vi "Periodic Tasks.vi"(8 "error in":errorcluster) -> ()   [LabVIEW 2012]
doc: "This VI runs in parallel to other tasks. It can contain as many user-defined periodic loops as you need. These can carry out PID or other sorts of timed response."
uses:
  <vilib>/Rock Robotics/SystemInterfaces/Utilities/FPGA_UtilitiesLED Source.ctl
  <vilib>/Rock Robotics/SystemInterfaces/Utilities/FPGA_UtilitiesLED State.ctl
  <vilib>/Rock Robotics/WPI/Compressor/WPI_CompressorGetSetRefNum.vi
  Robot Global Data.vi
  <vilib>/Rock Robotics/WPI/Joystick/WPI_JoystickGetSetRefNum.vi
  <vilib>/Rock Robotics/WPI/RobotDrive/WPI_RobotDriveGetSetRefNum.vi
panel:
  out "Current angle (deg) Right":dbl(knob) scale=0.0..360.0
  out "Distance (in) Right":dbl
  out "Revolutions Right":dbl
  out "Encoder Rate (in/sec) Right":dbl
  out "Encoder Status Right":string
  out "Encoder Direction Right":string
  out "Current angle (deg) Left":dbl(knob) scale=0.0..360.0
  out "Distance (in) Left":dbl
  out "Revolutions Left":dbl
  out "Encoder Rate (in/sec) Left":dbl
  out "Encoder Status Left":string
  out "Encoder Direction Left":string
  in  "Wheel dia. (in)":dbl=6.0
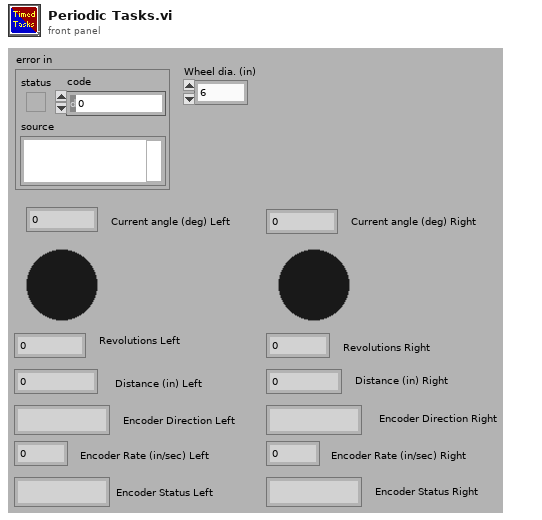
[diagram p1: front panel]
types:
  T1 = typedef "WPI_JoystickDevRef.ctl" = cluster{"Device":T2}
  T2 = typedef "WPI_JoystickDeviceEnum.ctl" = enum16{"USB 1", "USB 2", "USB 3", "USB 4", "Kinect 1", "Kinect 2"}
  T3 = typedef "WPI_RobotDriveDevRef.ctl" = cluster{"DevStatus":errorcluster, "Motors[]":T4[], "Square Inputs":bool, "Max Output":dbl, "Isochronous":bool}
  T4 = typedef "WPI_MotorControlDeviceRef.ctl" = cluster{"DeviceStatus":errorcluster, "Type":enum16{"PWM", "CAN"}, "PWM":cluster{"Digital Module":T5, "PWM Channel":T6, "DeadBand":T7}, "CAN":cluster{"Device Number":u8, "Control Mode":T8, "Semaphore":T9, "Max Vout":dbl}, "Invert":bool, "TransformRef":T10, "InvTransformRef":T10}
  T5 = typedef "FPGA_TypedefDigitalModule.ctl" = enum16{"Digital Module 1", "Digital Module 2"}
  T6 = typedef "FPGA_DIOPWMChannel.ctl" = enum8{"PWM 1", "PWM 2", "PWM 3", "PWM 4", "PWM 5", "PWM 6", "PWM 7", "PWM 8", "PWM 9", "PWM 10", "Invalid"}
  T7 = typedef "WPI_PWMDeadband.ctl" = cluster{"Name":string, "maxPositivePwm":i32, "minPositivePwm":i32, "centerPwm":i32, "maxNegativePwm":i32, "minNegativePwm":i32, "angularRange":u16}
  T8 = typedef "WPI_CANJaguar_ControlMode.ctl" = enum8{"Percent VBus", "Current", "Speed", "Position", "Voltage"}
  T9 = typedef "Semaphore RefNum" = refnum<k1>
  T10 = typedef "WPI_PWMTransform_ConPane.ctl" = refnum<vi>
  T11 = typedef "WPI_EncoderDevRef.ctl" = cluster{"DevStatus":errorcluster, "EncoderIndex":T12, "CounterIndex":T13, "DistancePerCount":dbl, "Decoding Type":T14}
  T12 = typedef "FPGA_EncoderIdx.ctl" = enum8{"Enc 0", "Enc 1", "Enc 2", "Enc 3", "Invalid"}
  T13 = typedef "FPGA_CounterCtrSystemIndex.ctl" = enum8{"Ctr 0", "Ctr 1", "Ctr 2", "Ctr 3", "Ctr 4", "Ctr 5", "Ctr 6", "Ctr 7", "Invalid"}
  T14 = typedef "WPI_EncoderType.ctl" = enum16{"1x", "2x", "4x"}
  T15 = cluster{"JoystickDevRef":T1, "RobotDriveDevRef":T3}
  T16 = typedef "FPGA_UtilitiesLED State.ctl" = enum16{"Off", "On", "Toggle"}
  T17 = typedef "FPGA_UtilitiesLED Source.ctl" = enum16{"User LED", "FPGA LED"}
  T18 = typedef "WPI_CompressorDevRef.ctl" = cluster{"DevStatus":errorcluster, "DigitalInputDevRef":T19, "RelayDevRef":T21}
  T19 = typedef "WPI_DigitalInputDevRef.ctl" = cluster{"DevStatus":errorcluster, "DIO Channel":T20, "Digital Module":T5}
  T20 = typedef "FPGA_DIOChannel.ctl" = enum8{"DIO 1", "DIO 2", "DIO 3", "DIO 4", "DIO 5", "DIO 6", "DIO 7", "DIO 8", "DIO 9", "DIO 10", "DIO 11", "DIO 12", "DIO 13", "DIO 14", "Invalid"}
  T21 = typedef "WPI_RelayDevRef.ctl" = cluster{"DevStatus":errorcluster, "Relay Channel":T22, "Digital Module":T5, "Relay Direction":T23}
  T22 = typedef "FPGA_DIORelayChannel.ctl" = enum8{"Relay 1", "Relay 2", "Relay 3", "Relay 4", "Relay 5", "Relay 6", "Relay 7", "Relay 8", "Invalid"}
  T23 = typedef "WPI_RelayDirection.ctl" = enum16{"Both directions", "Forward only", "Reverse only"}
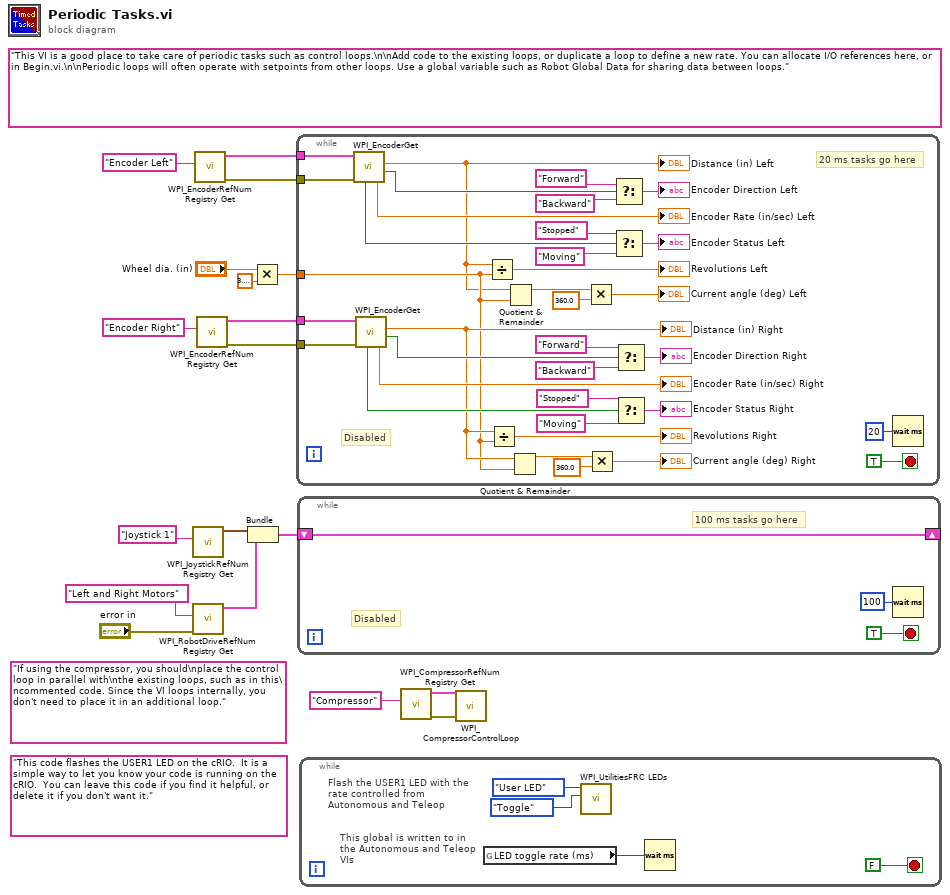
[diagram p0: block diagram]
diagram:
  (unwired) "If using the compressor, you should\nplace the control loop in parallel with\nthe existing loops, such as in this\ncommented code. Since the VI loops internally, you don't need to place it in an additional loop."
  (unwired) "This code flashes the USER1 LED on the cRIO.  It is a simple way to let you know your code is running on the cRIO.  You can leave this code if you find it helpful, or delete it if you don't want it."
  (unwired) "This VI is a good place to take care of periodic tasks such as control loops.\n\nAdd code to the existing loops, or duplicate a loop to define a new rate. You can allocate I/O references here, or in Begin.vi.\n\nPeriodic loops will often operate with setpoints from other loops. Use a global variable such as Robot Global Data for sharing data between loops."
  n1 = call <vilib>:"WPI_JoystickRefNum Registry Get.vi"("refnum name"="Joystick 1") -> ("JoystickDevRef"=w16:T1)  [unwired: 1 in, 9 out]
  n2 = call <vilib>:"WPI_RobotDriveRefNum Registry Get.vi"("error in (no error)"="error in", "refnum name"="Left and Right Motors") -> ("RobotDriveDevRef"=w15:T3)  [unwired: 9 out]
  n3 = call <vilib>:"WPI_EncoderRefNum Registry Get.vi"("refnum name"="Encoder Left") -> ("error out"=w9:errorcluster, "EncoderDevRef"=w10:T11)  [unwired: 9 in]
  n4 = call <vilib>:"WPI_EncoderRefNum Registry Get.vi"("refnum name"="Encoder Right") -> ("error out"=w7:errorcluster, "EncoderDevRef"=w8:T11)  [unwired: 9 in]
  n5 = Bundle("JoystickDevRef"=w16, "RobotDriveDevRef"=w15) -> (w14:T15)  [unwired: 1 out]
  n6 = Multiply(x="Wheel dia. (in)", y=3.141592653589793) -> (x*y=w4:dbl)
  n7 = while {
    tunnel: w10 -> [w34]
    tunnel: w9 -> [w33]
    tunnel: w8 -> [w29]
    tunnel: w7 -> [w28]
    tunnel: w4 -> [w26]
    stop <- TRUE stop-if-true
    # "Disabled"
    # "20 ms tasks go here"
    n8 = call <vilib>:"WPI_EncoderGet.vi"("error in (no error)"=w33, "EncoderDevRef"=w34) -> ("Direction"=w37:bool, "Distance"=w25:dbl, "Rate"=→"Encoder Rate (in/sec) Left":dbl, "Stopped"=w35:bool)  [unwired: 6 out]
    "Distance (in) Left" <- w25
    n9 = call <vilib>:"WPI_EncoderGet.vi"("error in (no error)"=w28, "EncoderDevRef"=w29) -> ("Direction"=w32:bool, "Distance"=w27:dbl, "Rate"=→"Encoder Rate (in/sec) Right":dbl, "Stopped"=w31:bool)  [unwired: 6 out]
    "Distance (in) Right" <- w27
    n10 = Divide(x=w25, y=w26) -> (x/y=→"Revolutions Left":dbl)
    n11 = Divide(x=w27, y=w26) -> (x/y=→"Revolutions Right":dbl)
    n12 = Quotient & Remainder(x=w25, y=w26) -> (x-y*floor(x/y)=w24:dbl)  [unwired: 1 out]
    n13 = Quotient & Remainder(x=w27, y=w26) -> (x-y*floor(x/y)=w20:dbl)  [unwired: 1 out]
    n14 = Multiply(x=w24, y=360.0) -> (x*y=→"Current angle (deg) Left":dbl)
    n15 = Multiply(x=w20, y=360.0) -> (x*y=→"Current angle (deg) Right":dbl)
    n16 = Select(t="Forward", s=w37, f="Backward") -> (s? t:f=→"Encoder Direction Left":string)
    n17 = Select(t="Stopped", s=w35, f="Moving") -> (s? t:f=→"Encoder Status Left":string)
    n18 = Select(t="Forward", s=w32, f="Backward") -> (s? t:f=→"Encoder Direction Right":string)
    n19 = Select(t="Stopped", s=w31, f="Moving") -> (s? t:f=→"Encoder Status Right":string)
    n20 = Wait (ms)(milliseconds to wait=u32 20) -> ()  [unwired: 1 out]
  }
  n21 = while {
    shift-right: [w54] -> _
    shift-left: w14 -> [w54]
    stop <- TRUE stop-if-true
    # "Disabled"
    # "100 ms tasks go here"
    n22 = Wait (ms)(milliseconds to wait=u32 100) -> ()  [unwired: 1 out]
  }
  n23 = while {
    stop <- FALSE stop-if-true
    # "This global is written to in the Autonomous and Teleop VIs"
    # "Flash the USER1 LED with the rate controlled from Autonomous and Teleop"
    n24 = global read "Robot Global Data.vi" "LED toggle rate (ms)"() -> (w57:u32)
    n25 = call <vilib>:"WPI_UtilitiesFRC LEDs.vi"("State"=FPGA_UtilitiesLED_State."Toggle", "LED Type"=FPGA_UtilitiesLED_Source."User LED") -> ()  [unwired: 1 in, 9 out]
    n26 = Wait (ms)(milliseconds to wait=w57) -> ()  [unwired: 1 out]
  }
  n27 = call <vilib>:"WPI_CompressorRefNum Registry Get.vi"("refnum name"="Compressor") -> ("error out"=w1:errorcluster, "CompressorDevRef"=w3:T18)  [unwired: 9 in]
  n28 = call <vilib>:"WPI_CompressorControlLoop.vi"("error in (no error)"=w1, "CompressorDevRef"=w3) -> ()  [unwired: 10 in]
